vi "Servo_SetAngle.vi"(9 "x":dbl min=-45.0 max=45.0, 10 "PWM":T1=1 items=["Invalid"=0, "PWM1"=1, "PWM2"=2, "PWM9"=9, "PWM10"=10]) -> (0 "error out":errorcluster, 3 "FPGA_Ref_out":refnum<k20>)   [LabVIEW 2009, in "Servo.lvlib"]
uses:
  Servo.lvlib
  PWM/PWM_Name.ctl
  PWM.lvlib
  FPGA.lvlib
panel:
  out "unsigned 32bit integer":u32
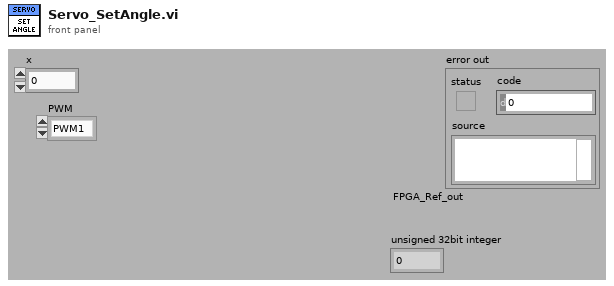
[diagram p1: front panel]
types:
  T1 = typedef "PWM.lvlib/PWM_Name.ctl" = u16
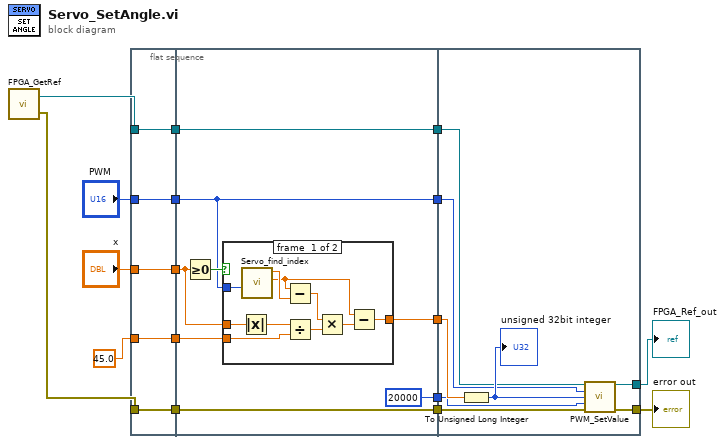
[diagram p0: block diagram]
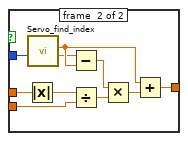
[diagram p2: hidden frame]
diagram:
  n1 = call "FPGA_GetRef.vi"() -> ("error out"=w1:errorcluster, "FPGA_Ref"=w2:refnum<k20>)  [unwired: 2 in]
  n2 = flat-sequence {
    tunnel: "PWM" -> [w21]
    tunnel: "x" -> [w22]
    tunnel: [w22] -> w17
    tunnel: [w21] -> w16
    tunnel: 45.0 ("y") -> [w20]
    tunnel: [w20] -> w15
    tunnel: w1 -> [w19]
    tunnel: [w19] -> w14
    tunnel: w2 -> [w18]
    tunnel: [w18] -> w13
    tunnel: w17 -> [w29]
    tunnel: w16 -> [w24]
    tunnel: [w28] -> w12
    tunnel: w15 -> [w27]
    tunnel: [u32 20000 ("Period (uSec)")] -> w11
    tunnel: [w25] -> w10
    tunnel: w14 -> [w25]
    tunnel: [w24] -> w9
    tunnel: [w23] -> w8
    tunnel: w13 -> [w23]
    tunnel: w12 -> [w58]
    tunnel: w11 -> [w56]
    tunnel: w10 -> [w55]
    tunnel: [w54] -> w5
    tunnel: w9 -> [w53]
    tunnel: w8 -> [w52]
    tunnel: [w51] -> w4
    frame #0 {
    }
    frame #1 {
      n3 = Greater Or Equal To 0?(x=w29) -> (x >= 0?=w30:bool)
      n4 = case shown="True" w30 {
        tunnel: w29 -> [w39 w49]
        tunnel: w24 -> [w40 w50]
        tunnel: [w36 w44] -> w28
        tunnel: w27 -> [w32 w46]
        frame #0 {
          n5 = Absolute Value(x=w39) -> (abs(x)=w33:dbl)
          n6 = call "Servo_find_index.vi"("PWM"=w40) -> ("value 2"=w34:dbl, "value"=w37:dbl)  [unwired: 7 in, 2 out]
          n7 = Subtract(x=w34, y=w37) -> (x-y=w38:dbl)
          n8 = Divide(x=w33, y=w32) -> (x/y=w31:dbl)
          n9 = Multiply(x=w38, y=w31) -> (x*y=w35:dbl)
          n10 = Subtract(x=w34, y=w35) -> (x-y=w36:dbl)
        }
        frame #1 {
          n11 = Absolute Value(x=w49) -> (abs(x)=w47:dbl)
          n12 = call "Servo_find_index.vi"("PWM"=w50) -> ("value 3"=w41:dbl, "value 2"=w42:dbl)  [unwired: 7 in, 2 out]
          n13 = Subtract(x=w41, y=w42) -> (x-y=w48:dbl)
          n14 = Divide(x=w47, y=w46) -> (x/y=w45:dbl)
          n15 = Multiply(x=w48, y=w45) -> (x*y=w43:dbl)
          n16 = Add(x=w42, y=w43) -> (x+y=w44:dbl)
        }
      }
    }
    frame #2 {
      n17 = To Unsigned Long Integer(number=w58) -> (unsigned 32bit integer=w57:u32)
      "unsigned 32bit integer" <- w57
      n18 = call "PWM_SetValue.vi"("FPGA_Ref_in"=w52, "PWM"=w53, "High (uSec)"=w57, "Period (uSec)"=w56, "error in"=w55) -> ("FPGA_Ref_out"=w51:refnum<k20>, "error out"=w54:errorcluster)  [unwired: 9 in]
    }
  }
  "error out" <- w5
  "FPGA_Ref_out" <- w4
